vi "Main.vi"(8 "error in (no error)":errorcluster, 11 "BMCBase in":refnum<class "BMC.lvclass">) -> (0 "error out":errorcluster, 3 "component":refnum<class "BMC.lvclass">)   [LabVIEW 2012, in "BMC.lvclass"]
doc: "Main VI of the component."
uses:
  BMC.lvclass
  <vilib>/Distrio/Murmex/Murmex/command_enum.ctl
  <vilib>/Distrio/Murmex/InitialiseMessage/InitialiseMessage.lvclass
  BMC.lvclass/BMC.ctl
  <vilib>/Distrio/Murmex/ResetMessage/ResetMessage.lvclass
  <vilib>/Distrio/Murmex/GenericMessage/GenericMessage.lvclass
  <vilib>/Distrio/Murmex/ConfigureMessage/ConfigureMessage.lvclass
  <vilib>/Distrio/Murmex/TerminateMessage/TerminateMessage.lvclass
  <vilib>/Distrio/Murmex/Murmex/update_cluster.ctl
  <vilib>/Distrio/Murmex/Murmex/Set configure at initialise.vi
  <vilib>/Distrio/Murmex/Murmex/Set log reference.vi
  <vilib>/Distrio/Murmex/Murmex/Set VI reference.vi
  <vilib>/Distrio/Murmex/Murmex/Get ID.vi
  <vilib>/Distrio/Murmex/Message/Add or replace parameter.vi
  <vilib>/Distrio/Murmex/Murmex/Murmex.lvclass
  <vilib>/Distrio/Murmex/Message/Message.lvclass
panel:
  in  "Tab Control":T1(tab)
  in  "button: resettomid":bool
  in  "Superactuator":dbl(knob)=50.0 min=0.0 max=300.0 step=1.0 scale=0.0..300.0
  in  "Mirror shape name":string="bob"
  in  "apply superactuator":bool
  in  "apply shape":bool
  in  "button:saveshape":bool
  in  "button: resettoflat":bool
  in  "Load Voltage file":path=path "D:/CLSM_Project/BMC/TestMap1.txt"
  out "DM Voltage Map":dbl[][](graph)
  out "Actuator stats":dbl[][](graph)
  out "log":string
  in  "Component id":string="BMC"
  in  "command":T2
  in  "button:send command":bool
  in  "generic command":string
  in  "button:configure":bool
  in  "button:quit":bool
  out "terminate?":bool
  # "Load voltage map"
  # "Save settings"
  # "Superactuator"
  # "Resets"
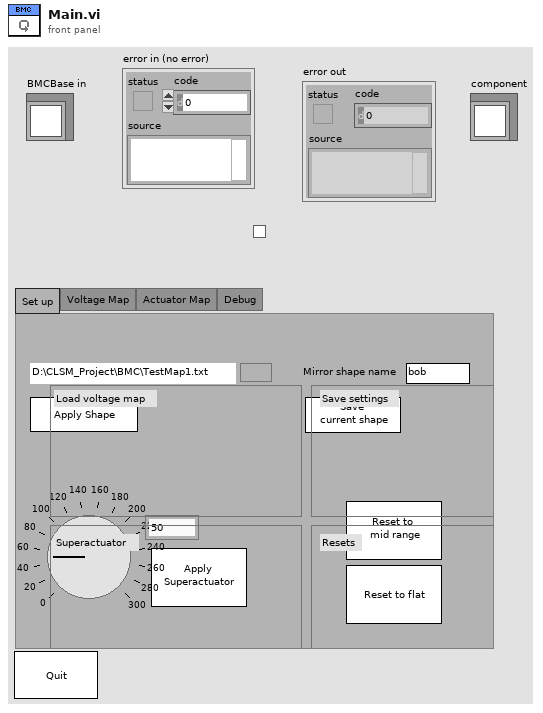
[diagram p1: front panel]
types:
  T1 = enum32{"Set up", "Voltage Map", "Actuator Map", "Debug"}
  T2 = typedef "Murmex.lvlib/Murmex.lvclass/command_enum.ctl" = enum16{"null", "initialise", "reset", "terminate", "acknowledge", "update", "inspect", "inform", "proceed", "start", "stop", "fetch", "configure", "generic"}
  T3 = enum8{"Enabled", "Disabled", "Disabled and Grayed Out"}
  T4 = typedef "Murmex.lvlib/Murmex.lvclass/update_cluster.ctl" = cluster{"target ID":string, "key chains":string[], "values":variant[]}
  T5 = typedef "Murmex.lvclass/command_enum.ctl" = enum16{"null", "initialise", "reset", "terminate", "acknowledge", "update", "inspect", "inform", "proceed", "start", "stop", "fetch", "configure", "generic"}
  T6 = typedef "Murmex.lvclass/Event type enumerations.ctl" = enum16{"before", "after"}
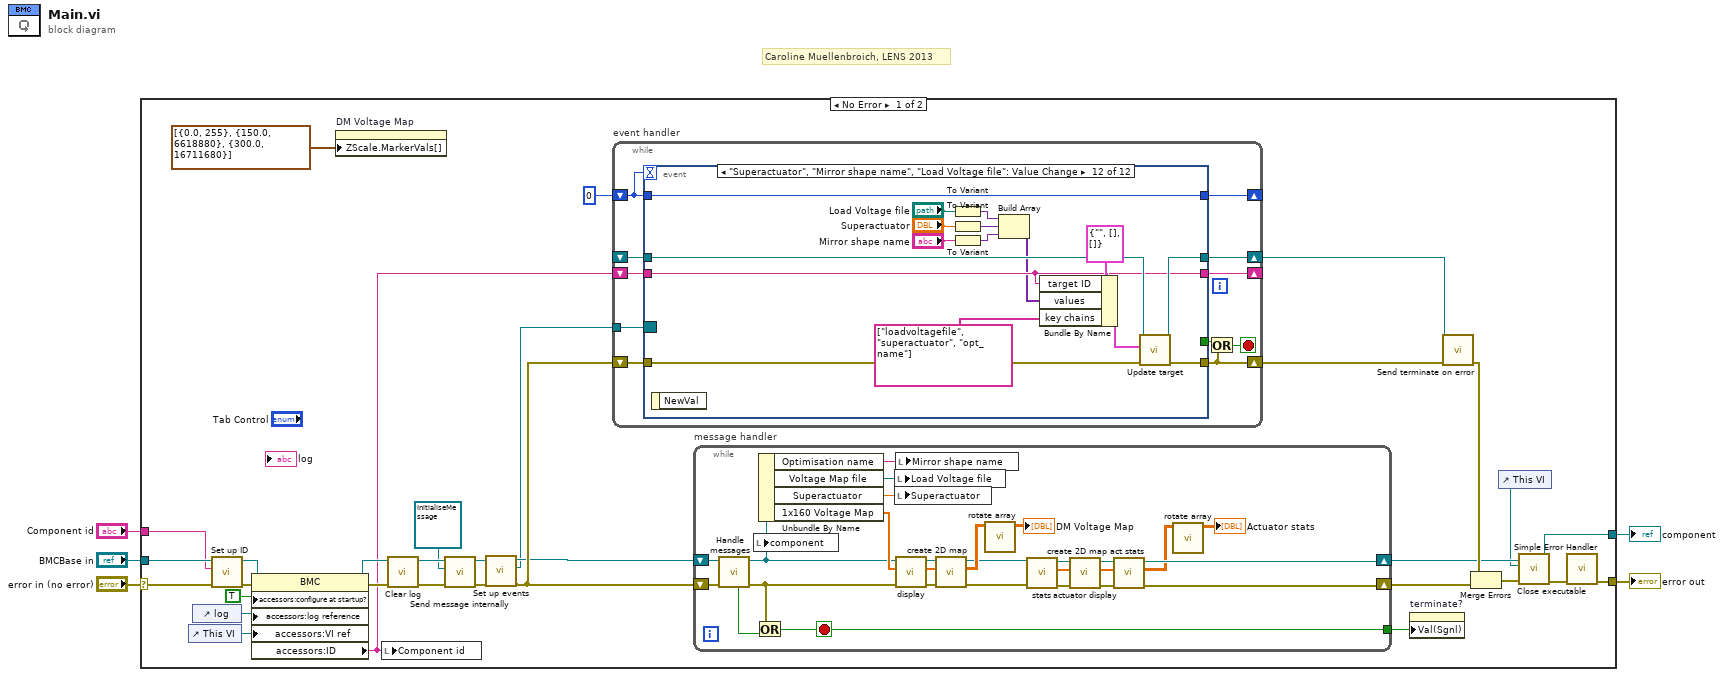
[diagram p0: block diagram]
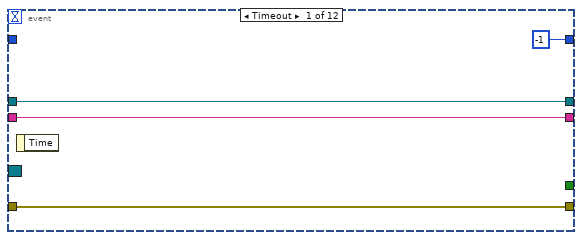
[diagram p2: hidden frame]
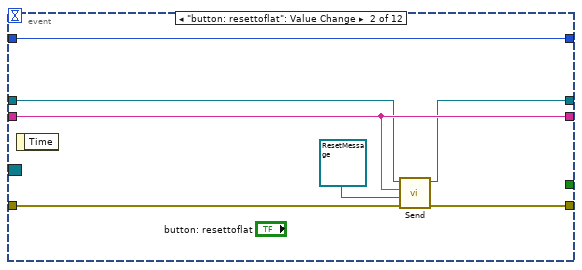
[diagram p3: hidden frame]
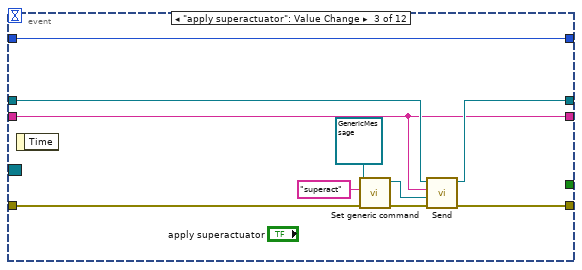
[diagram p4: hidden frame]
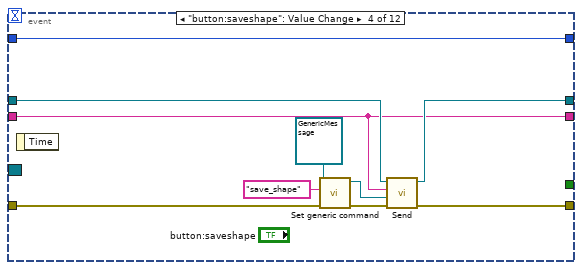
[diagram p5: hidden frame]
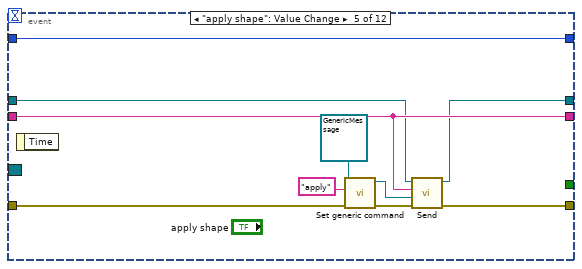
[diagram p6: hidden frame]
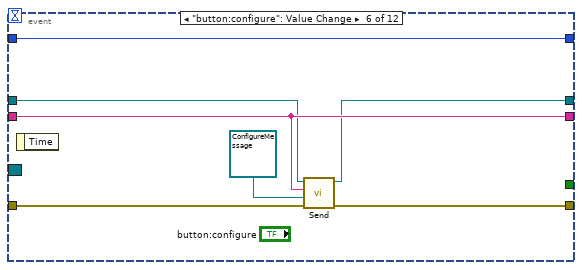
[diagram p7: hidden frame]
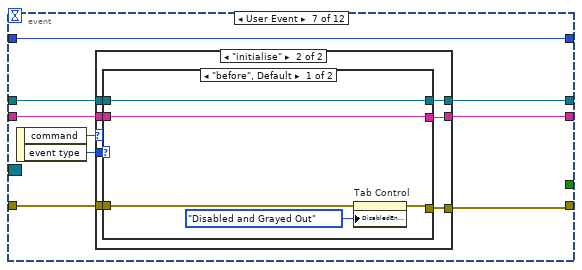
[diagram p8: hidden frame]
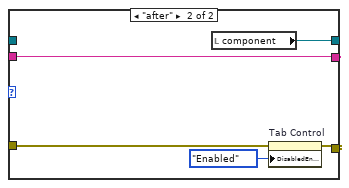
[diagram p10: hidden frame]
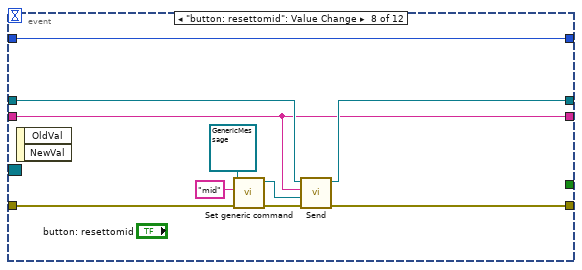
[diagram p11: hidden frame]
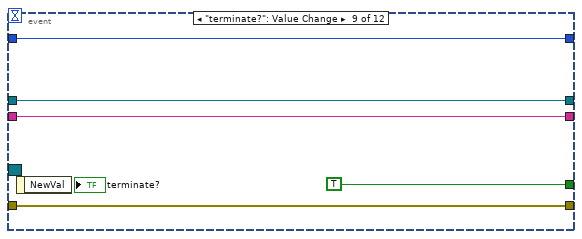
[diagram p12: hidden frame]
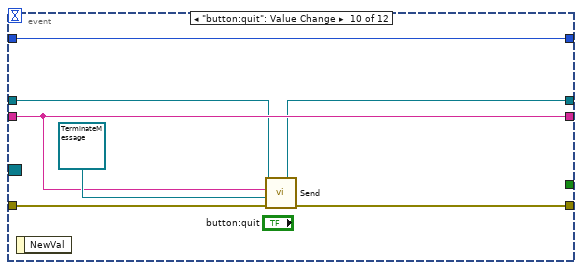
[diagram p13: hidden frame]
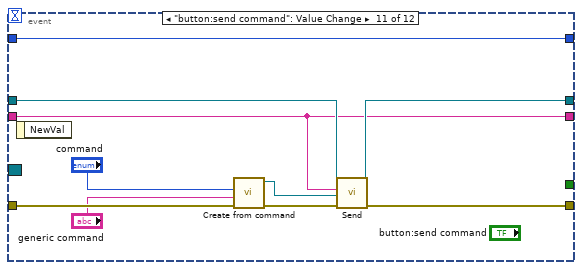
[diagram p14: hidden frame]
diagram:
  # "Caroline Muellenbroich, LENS 2013"
  n1 = case shown="No Error" "error in (no error)" {
    selector: "error in (no error)" -> [w23 w202]
    tunnel: [w8 w201] -> w5
    tunnel: "BMCBase in" -> [w27 w201]
    tunnel: [w9 w202] -> w3
    tunnel: "Component id" -> [w22 _]
    frame No Error {
      n2 = control-ref of="This VI"() -> (w34:refnum<vi>)
      n3 = control-ref of="log"() -> (w35:refnum<vi>)
      n4 = call <vilib>:"Set up ID.vi"("error in (no error)"=w23, "component ID"=w22, "MurmexBase in"=w27) -> ("error out"=w28:errorcluster, "MurmexBase out"=w26:refnum<class "BMC.lvclass">)  [unwired: 6 in, 1 out]
      n5 = property class="BMC"(reference=w26, error in=w28, "accessors:configure at startup?"=TRUE ("configure at startup?"), "accessors:log reference"=w35, "accessors:VI ref"=w34) -> (reference out=w37:refnum<class "BMC.lvclass">, error out=w32:errorcluster, "accessors:ID"=w15:string)
      n6 = property on="DM Voltage Map" class="IntGraph (strict)"("ZScale.MarkerVals[]"=cluster{dbl, u32}[] [{0.0, 255}, {150.0, 6618880}, {300.0, 16711680}] ("Z Scale.Marker Values[]")) -> ()  [unwired: 2 in, 2 out]
      n7 = local write "Component id"(w15) -> ()
      n8 = call <vilib>:"Clear log.vi"("error in (no error)"=w32, "MurmexBase in"=w37) -> ("error out"=w31:errorcluster, "MurmexBase out"=w33:refnum<class "BMC.lvclass">)  [unwired: 8 in]
      n9 = call <vilib>:"Send message internally.vi"("error in (no error)"=w31, "Message"=refnum<class "InitialiseMessage.lvclass"> refnum ("InitialiseMessage"), "Murmex in"=w33) -> ("error out"=w21:errorcluster, "Murmex out"=w19:refnum<class "BMC.lvclass">)  [unwired: 7 in]
      n10 = call <vilib>:"Set up events.vi"("error in (no error)"=w21, "MurmexBase in"=w19) -> ("error out"=w20:errorcluster, "Event Registration Refnum"=w17:refnum<event-registration>, "MurmexBase out"=w18:refnum<class "BMC.lvclass">)  [unwired: 7 in]
      n11 = while "event handler" {
        shift-right: [w47] -> w14
        shift-left: w20 -> [w48]
        tunnel: w17 -> [w44]
        shift-right: [w42] -> _
        shift-left: 0 -> [w43]
        shift-right: [w40] -> _
        shift-left: w15 -> [w41]
        shift-right: [w39] -> w12
        shift-left: _ -> [w38]
        stop <- w45 stop-if-true
        n12 = event shown="[11] \"Superactuator\", \"Mirror shape name\", \"Load Voltage file\": Value Change" {
          selector: w44 -> [_ _ _ _ _ _ _ _ _ _ _ _]
          dyn-events: _ -> [_ _ _ _ _ _ _ _ _ _ _ _]
          timeout: w43 -> [_ _ _ _ _ _ _ _ _ _ _ _]
          tunnel: w48 -> [w52 w54 w64 w75 w85 w96 w103 w128 w140 w145 w157 w171]
          tunnel: [w52 w58 w65 w74 w84 w95 w98 w127 w140 w147 w155 w170] -> w47
          tunnel: [_ _ _ _ _ _ _ _ TRUE _ _ _] -> w46
          tunnel: w43 -> [_ w59 w60 w70 w80 w92 w97 w131 w136 w141 w148 w164]
          tunnel: [-1 w59 w60 w70 w80 w92 w97 w131 w136 w141 w148 w164] -> w42
          tunnel: w41 -> [w50 w57 w61 w71 w83 w93 w102 w126 w138 w144 w149 w166]
          tunnel: [w50 w57 w61 w71 w83 w93 w101 w126 w138 w144 w149 w166] -> w40
          tunnel: [w49 w55 w62 w72 w82 w90 w100 w129 w137 w142 w150 w168] -> w39
          tunnel: w38 -> [w49 w56 w63 w73 w81 w91 w99 w130 w137 w143 w151 w169]
          event Timeout {
            n13 = event-data() -> ()  [unwired: 1 in, 1 out]
          }
          event "button: resettoflat": Value Change {
            n14 = event-data() -> ()  [unwired: 1 in, 1 out]
            n15 = call <vilib>:"Send.vi"("error in (no error)"=w54, "Message"=refnum<class "ResetMessage.lvclass"> refnum ("Message in"), "recipient"=w57, "Murmex in"=w56) -> ("error out"=w58:errorcluster, "Murmex out"=w55:refnum<class "Murmex.lvclass">)  [unwired: 6 in]
          }
          event "apply superactuator": Value Change {
            n16 = event-data() -> ()  [unwired: 1 in, 1 out]
            n17 = call <vilib>:"Set generic command.vi"("error in (no error)"=w64, "generic command"="superact", "GenericMessage in"=refnum<class "GenericMessage.lvclass"> refnum ("GenericMessage")) -> ("error out"=w68:errorcluster, "GenericMessage out"=w67:refnum<class "GenericMessage.lvclass">)  [unwired: 7 in]
            n18 = call <vilib>:"Send.vi"("error in (no error)"=w68, "Message"=w67, "recipient"=w61, "Murmex in"=w63) -> ("error out"=w65:errorcluster, "Murmex out"=w62:refnum<class "Murmex.lvclass">)  [unwired: 6 in]
          }
          event "button:saveshape": Value Change {
            n19 = event-data() -> ()  [unwired: 1 in, 1 out]
            n20 = call <vilib>:"Set generic command.vi"("error in (no error)"=w75, "generic command"="save_shape", "GenericMessage in"=refnum<class "GenericMessage.lvclass"> refnum ("GenericMessage")) -> ("error out"=w78:errorcluster, "GenericMessage out"=w77:refnum<class "GenericMessage.lvclass">)  [unwired: 7 in]
            n21 = call <vilib>:"Send.vi"("error in (no error)"=w78, "Message"=w77, "recipient"=w71, "Murmex in"=w73) -> ("error out"=w74:errorcluster, "Murmex out"=w72:refnum<class "Murmex.lvclass">)  [unwired: 6 in]
          }
          event "apply shape": Value Change {
            n22 = event-data() -> ()  [unwired: 1 in, 1 out]
            n23 = call <vilib>:"Set generic command.vi"("error in (no error)"=w85, "generic command"="apply", "GenericMessage in"=refnum<class "GenericMessage.lvclass"> refnum ("GenericMessage")) -> ("error out"=w88:errorcluster, "GenericMessage out"=w87:refnum<class "GenericMessage.lvclass">)  [unwired: 7 in]
            n24 = call <vilib>:"Send.vi"("error in (no error)"=w88, "Message"=w87, "recipient"=w83, "Murmex in"=w81) -> ("error out"=w84:errorcluster, "Murmex out"=w82:refnum<class "Murmex.lvclass">)  [unwired: 6 in]
          }
          event "button:configure": Value Change {
            n25 = event-data() -> ()  [unwired: 1 in, 1 out]
            n26 = call <vilib>:"Send.vi"("error in (no error)"=w96, "Message"=refnum<class "ConfigureMessage.lvclass"> refnum ("ConfigureMessage"), "recipient"=w93, "Murmex in"=w91) -> ("error out"=w95:errorcluster, "Murmex out"=w90:refnum<class "Murmex.lvclass">)  [unwired: 6 in]
          }
          event User Event {
            n27 = event-data() -> ("command"=w105:T5, "event type"=w104:T6)  [unwired: 1 in]
            n28 = case shown="\"initialise\"" w105 {
              tunnel: w104 -> [_ w115]
              tunnel: w103 -> [w106 w114]
              tunnel: w102 -> [w107 w113]
              tunnel: [w107 w112] -> w101
              tunnel: [w108 w111] -> w100
              tunnel: w99 -> [w108 w110]
              tunnel: [w106 w109] -> w98
              frame "null", Default {
              }
              frame "initialise" {
                n29 = case shown="\"before\", Default" w115 {
                  tunnel: w114 -> [w117 w125]
                  tunnel: [w116 w123] -> w109
                  tunnel: [w119 w122] -> w112
                  tunnel: w113 -> [w119 w122]
                  tunnel: [w120 w121] -> w111
                  tunnel: w110 -> [w120 _]
                  frame "before", Default {
                    n30 = property on="Tab Control" class="TabCtl (strict)"(error in=w117, "DisabledEnum"=T3."Disabled and Grayed Out" ("Disabled")) -> (error out=w116:errorcluster)  [unwired: 1 in, 1 out]
                  }
                  frame "after" {
                    n31 = local read "component"() -> (w121:refnum<class "BMC.lvclass">)
                    n32 = property on="Tab Control" class="TabCtl (strict)"(error in=w125, "DisabledEnum"=T3."Enabled" ("Disabled")) -> (error out=w123:errorcluster)  [unwired: 1 in, 1 out]
                  }
                }
              }
            }
          }
          event "button: resettomid": Value Change {
            n33 = event-data() -> ()  [unwired: 1 in, 2 out]
            n34 = call <vilib>:"Set generic command.vi"("error in (no error)"=w128, "generic command"="mid", "GenericMessage in"=refnum<class "GenericMessage.lvclass"> refnum ("GenericMessage")) -> ("error out"=w133:errorcluster, "GenericMessage out"=w134:refnum<class "GenericMessage.lvclass">)  [unwired: 7 in]
            n35 = call <vilib>:"Send.vi"("error in (no error)"=w133, "Message"=w134, "recipient"=w126, "Murmex in"=w130) -> ("error out"=w127:errorcluster, "Murmex out"=w129:refnum<class "Murmex.lvclass">)  [unwired: 6 in]
          }
          event "terminate?": Value Change {
            n36 = event-data() -> ()  [unwired: 1 in, 1 out]
          }
          event "button:quit": Value Change {
            n37 = event-data() -> ()  [unwired: 1 in, 1 out]
            n38 = call <vilib>:"Send.vi"("error in (no error)"=w145, "Message"=refnum<class "TerminateMessage.lvclass"> refnum ("TerminateMessage"), "recipient"=w144, "Murmex in"=w143) -> ("error out"=w147:errorcluster, "Murmex out"=w142:refnum<class "Murmex.lvclass">)  [unwired: 6 in]
          }
          event "button:send command": Value Change {
            n39 = event-data() -> ()  [unwired: 1 in, 1 out]
            n40 = call <vilib>:"Create from command.vi"("error in (no error)"=w157, "generic command"="generic command", "command"="command") -> ("error out"=w152:errorcluster, "Message out"=w156:refnum<class "Message.lvclass">)  [unwired: 7 in]
            n41 = call <vilib>:"Send.vi"("error in (no error)"=w152, "Message"=w156, "recipient"=w149, "Murmex in"=w151) -> ("error out"=w155:errorcluster, "Murmex out"=w150:refnum<class "Murmex.lvclass">)  [unwired: 6 in]
          }
          event "Superactuator", "Mirror shape name", "Load Voltage file": Value Change {
            n42 = event-data() -> ()  [unwired: 1 in, 1 out]
            n43 = To Variant(anything="Load Voltage file") -> (Variant=w160:variant)
            n44 = To Variant(anything="Superactuator") -> (Variant=w161:variant)
            n45 = To Variant(anything="Mirror shape name") -> (Variant=w162:variant)
            n46 = Build Array(w160, w161, w162) -> (w165:variant[])
            n47 = Bundle By Name(cluster=T4 {"target ID"="", "key chains"=[], "values"=[]} ("update cluster"), "target ID"=w166, "values"=w165, "key chains"=string[] ["loadvoltagefile", "superactuator", "opt_name"]) -> (w172:T4)
            n48 = call <vilib>:"Update target.vi"("error in (no error)"=w171, "update cluster"=w172, "MurmexBase in"=w169) -> ("error out"=w170:errorcluster, "MurmexBase out"=w168:refnum<class "Murmex.lvclass">)  [unwired: 7 in]
          }
        }
        n49 = Or(x=w46, y=w47) -> (x .or. y?=w45:bool)
      }
      n50 = while "message handler" {
        shift-right: [w185] -> w25
        shift-left: w20 -> [w200]
        shift-right: [w181] -> w7
        shift-left: w18 -> [w197]
        tunnel: [w198] -> w29
        stop <- w198 stop-if-true
        n51 = call <vilib>:"Handle messages.vi"("error in (no error)"=w200, "Murmex in"=w197) -> ("error out"=w194:errorcluster, "Murmex out"=w177:refnum<class "BMC.lvclass">, "terminated?"=w199:bool)  [unwired: 7 in]
        n52 = local write "component"(w177) -> ()
        n53 = Or(x=w194, y=w199) -> (x .or. y?=w198:bool)
        n54 = Unbundle By Name(w177) -> ("Optimisation name"=w174:string, "Voltage Map file"=w175:path, "Superactuator"=w176:dbl, "1x160 Voltage Map"=w193:dbl[])
        n55 = local write "Load Voltage file"(w175) -> ()
        n56 = local write "Superactuator"(w176) -> ()
        n57 = local write "Mirror shape name"(w174) -> ()
        n58 = call "display.vi"("error in (no error)"=w194, "1x160 Voltage Map"=w193, "BMC in"=w177) -> ("error out"=w189:errorcluster, "1x160 Voltage Map 2"=w188:dbl[], "BMC out"=w190:refnum<class "BMC.lvclass">)  [unwired: 6 in]
        n59 = call-dynamic "create 2D map.vi"("error in (no error)"=w189, "Voltage array"=w188, "BMC in"=w190) -> ("error out"=w186:errorcluster, "2D Voltage Map"=w195:dbl[][], "BMC out"=w184:refnum<class "BMC.lvclass">)  [unwired: 6 in]
        n60 = call "rotate array.vi"("Array 2"=w195) -> ("Array"=→"DM Voltage Map":dbl[][])  [unwired: 10 in]
        n61 = call-dynamic "stats.vi"("error in (no error)"=w186, "BMC in"=w184) -> ("error out"=w192:errorcluster, "actuator array"=w191:dbl[], "BMC out"=w183:refnum<class "BMC.lvclass">)  [unwired: 7 in]
        n62 = call "actuator display.vi"("error in (no error)"=w192, "actuator array in"=w191, "BMC in"=w183) -> ("error out"=w187:errorcluster, "actuator array out"=w178:dbl[], "BMC out"=w182:refnum<class "BMC.lvclass">)  [unwired: 6 in]
        n63 = call-dynamic "create 2D map act stats.vi"("error in (no error)"=w187, "Actuator array in"=w178, "BMC in"=w182) -> ("error out"=w185:errorcluster, "actuator stats out"=w179:dbl[][], "BMC out"=w181:refnum<class "BMC.lvclass">)  [unwired: 6 in]
        n64 = call "rotate array.vi"("Array 2"=w179) -> ("Array"=→"Actuator stats":dbl[][])  [unwired: 10 in]
      }
      n65 = property on="terminate?" class="Bool (strict)"("Val(Sgnl)"=w29) -> ()  [unwired: 2 in, 2 out]
      n66 = call <vilib>:"Send terminate on error.vi"("error in (no error)"=w14, "Murmex in"=w12) -> ("error out"=w13:errorcluster)  [unwired: 8 in, 1 out]
      n67 = Merge Errors(w13, w25) -> (w10:errorcluster)
      n68 = control-ref of="This VI"() -> (w6:refnum<vi>)
      n69 = call <vilib>:"Close executable.vi"("error in (no error)"=w10, "main VI ref (optional)"=w6, "MurmexBase in"=w7) -> ("error out"=w11:errorcluster, "MurmexBase out"=w8:refnum<class "BMC.lvclass">)  [unwired: 7 in]
      n70 = call <vilib>:"Simple Error Handler.vi"("error in (no error)"=w11) -> ("error out"=w9:errorcluster)  [unwired: 4 in, 4 out]
    }
    frame Error {
    }
  }
  "error out" <- w3
  "component" <- w5
